vi "Separate Unacceptable pO2 Estimates.vi"(9 "All Times":dbl[](array[numeric]), 10 "All pO2 Estimates":dbl[][](array[numeric]), 11 "Oxy Unacceptable Estimate Flags":bool[](array[boolean])) -> (0 "Bad pO2 Estimates":dbl[][](array[numeric]), 1 "Bad pO2 Estimate Times":dbl[](array[numeric]), 2 "Good pO2 Estimates":dbl[][](array[numeric]), 3 "Good pO2 Estimate Times":dbl[](array[numeric]))   [LabVIEW 2016]
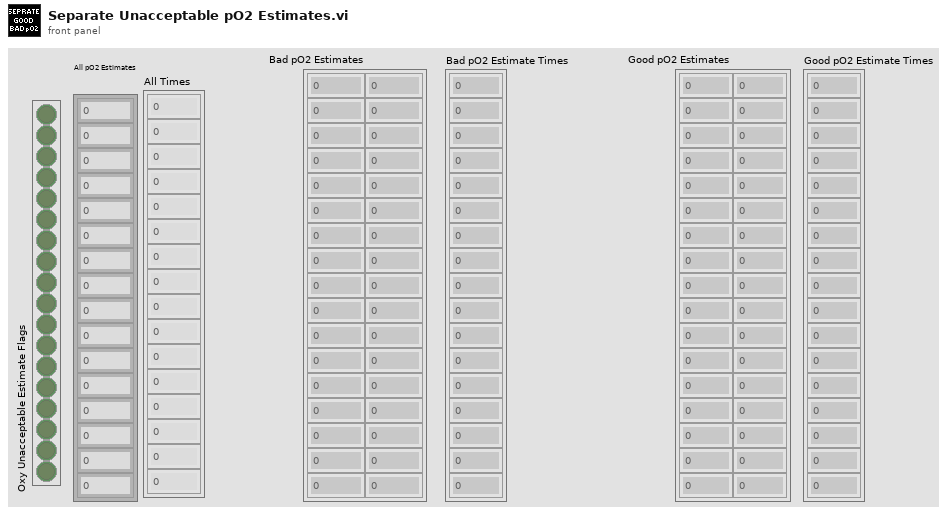
[diagram p1: front panel]
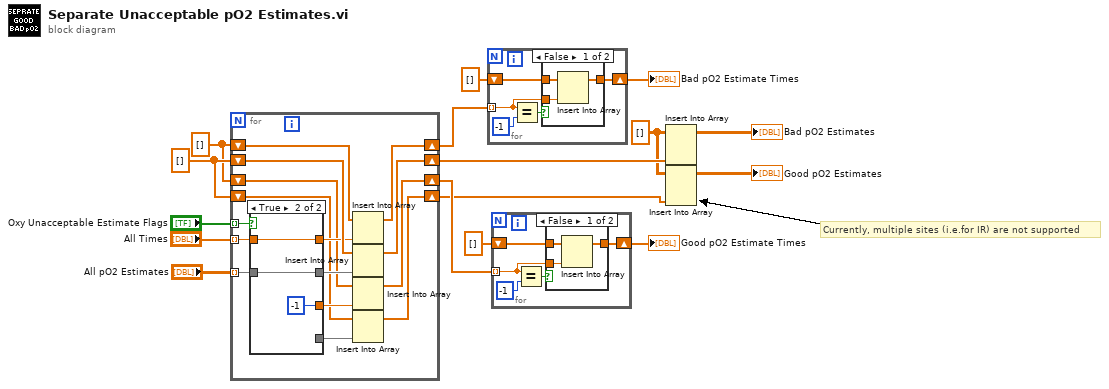
[diagram p0: block diagram]
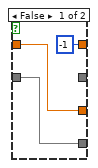
[diagram p4: hidden frame]
diagram:
  w3 = dbl[][] [] ("array")
  w12 = dbl[] []
  w13 = dbl[] []
  # "Currently, multiple sites (i.e.for IR) are not supported"
  n1 = for {
    tunnel: "Oxy Unacceptable Estimate Flags" -> [w31] mode=indexing
    tunnel: "All pO2 Estimates" -> [w30] mode=indexing
    tunnel: "All Times" -> [w29] mode=indexing
    shift-right: [w26] -> w5
    shift-left: w13 -> [w28]
    shift-right: [w24] -> w11
    shift-left: w12 -> [w21]
    shift-right: [w20] -> w8
    shift-left: w12 -> [w18]
    shift-right: [w19] -> w4
    shift-left: w13 -> [w17]
    n2 = case shown="True" w31 {
      tunnel: w30 -> [w33 w37]
      tunnel: w29 -> [w34 w36]
      tunnel: [_ w37] -> w27
      tunnel: [-1 w36] -> w25
      tunnel: [w34 -1] -> w23
      tunnel: [w33 _] -> w22
      frame False {
      }
      frame True {
      }
    }
    n3 = Insert Into Array(array=w21, new element=w25) -> (w24:dbl[])  [unwired: 1 in]
    n4 = Insert Into Array(array=w28, new element=w27) -> (w26:dbl[])  [unwired: 1 in]
    n5 = Insert Into Array(array=w18, new element=w23) -> (w20:dbl[])  [unwired: 1 in]
    n6 = Insert Into Array(array=w17, new element=w22) -> (w19:dbl[])  [unwired: 1 in]
  }
  n7 = for {
    tunnel: w11 -> [w40] mode=indexing
    shift-right: [w39] -> w9
    shift-left: dbl[] [] -> [w38]
    n8 = Equal?(x=w40, y=-1) -> (x = y?=w41:bool)
    n9 = case shown="False" w41 {
      tunnel: w40 -> [w44 _]
      tunnel: [w45 w46] -> w39
      tunnel: w38 -> [w43 w46]
      frame False {
        n10 = Insert Into Array(array=w43, new element=w44) -> (w45:dbl[])  [unwired: 1 in]
      }
      frame True {
      }
    }
  }
  "Bad pO2 Estimate Times" <- w9
  n11 = for {
    tunnel: w8 -> [w49] mode=indexing
    shift-right: [w48] -> w6
    shift-left: dbl[] [] -> [w47]
    n12 = Equal?(x=w49, y=-1) -> (x = y?=w50:bool)
    n13 = case shown="False" w50 {
      tunnel: w49 -> [w53 _]
      tunnel: [w54 w55] -> w48
      tunnel: w47 -> [w52 w55]
      frame False {
        n14 = Insert Into Array(array=w52, new element=w53) -> (w54:dbl[])  [unwired: 1 in]
      }
      frame True {
      }
    }
  }
  "Good pO2 Estimate Times" <- w6
  n15 = Insert Into Array(array=w3, new element=w5) -> (→"Bad pO2 Estimates":dbl[][])  [unwired: 2 in]
  n16 = Insert Into Array(array=w3, new element=w4) -> (→"Good pO2 Estimates":dbl[][])  [unwired: 2 in]
